vi "GVSView Pic Command Remove.vi"(10 "cCommand":T1) -> ()   [LabVIEW 2013]
uses:
  GVSView Global.vi
panel:
  out "Start_Positin 2":T2
  in  "ToolBar Click":bool
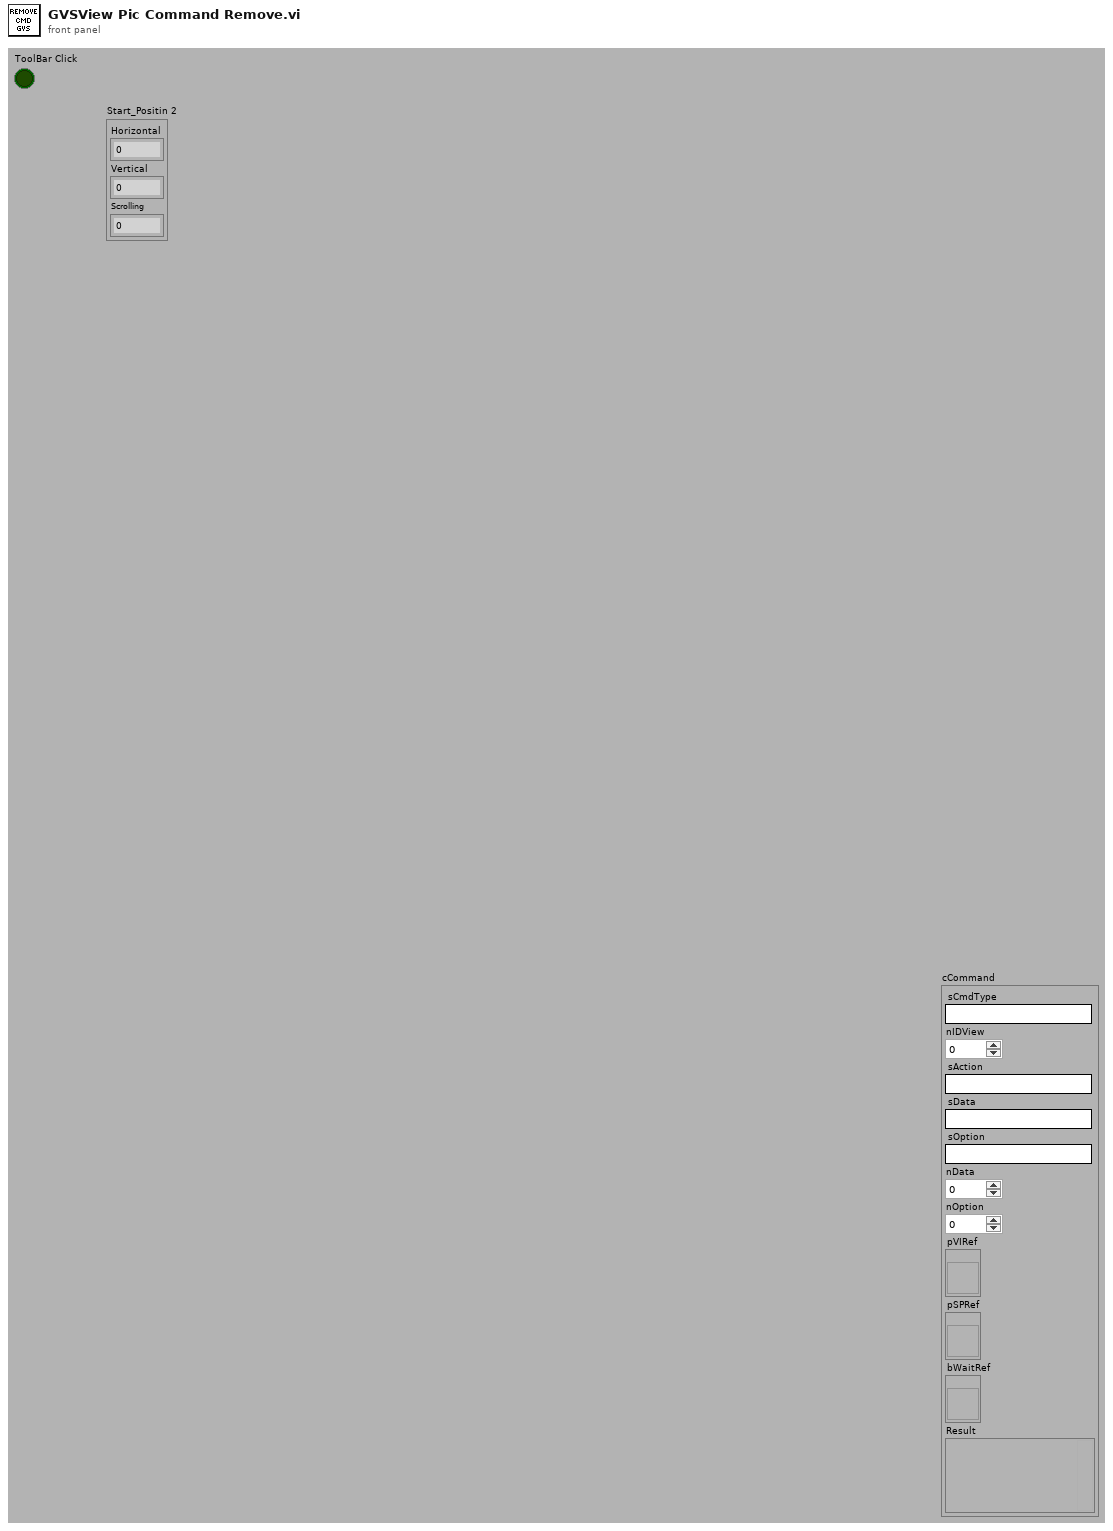
[diagram p1: front panel]
types:
  T1 = cluster{"sCmdType":string, "nIDView":i32, "sAction":string, "sData":string, "sOption":string, "nData":i32, "nOption":i32, "pVIRef":refnum<vi>, "pSPRef":refnum<vi>, "bWaitRef":refnum<vi>, "Result":variant}
  T2 = cluster{"Horizontal":i32, "Vertical":i32, "Scrolling":i32}
  T3 = cluster{"sCmdType":string, "nIDView":i32, "sAction":string, "sData":string, "sOption":string, "nData":i32, "nOption":i32, "pVIRef":refnum<vi>, "pSPRef":refnum<vi>, "bWaitRef":refnum<vi>, "Result":variant}[]
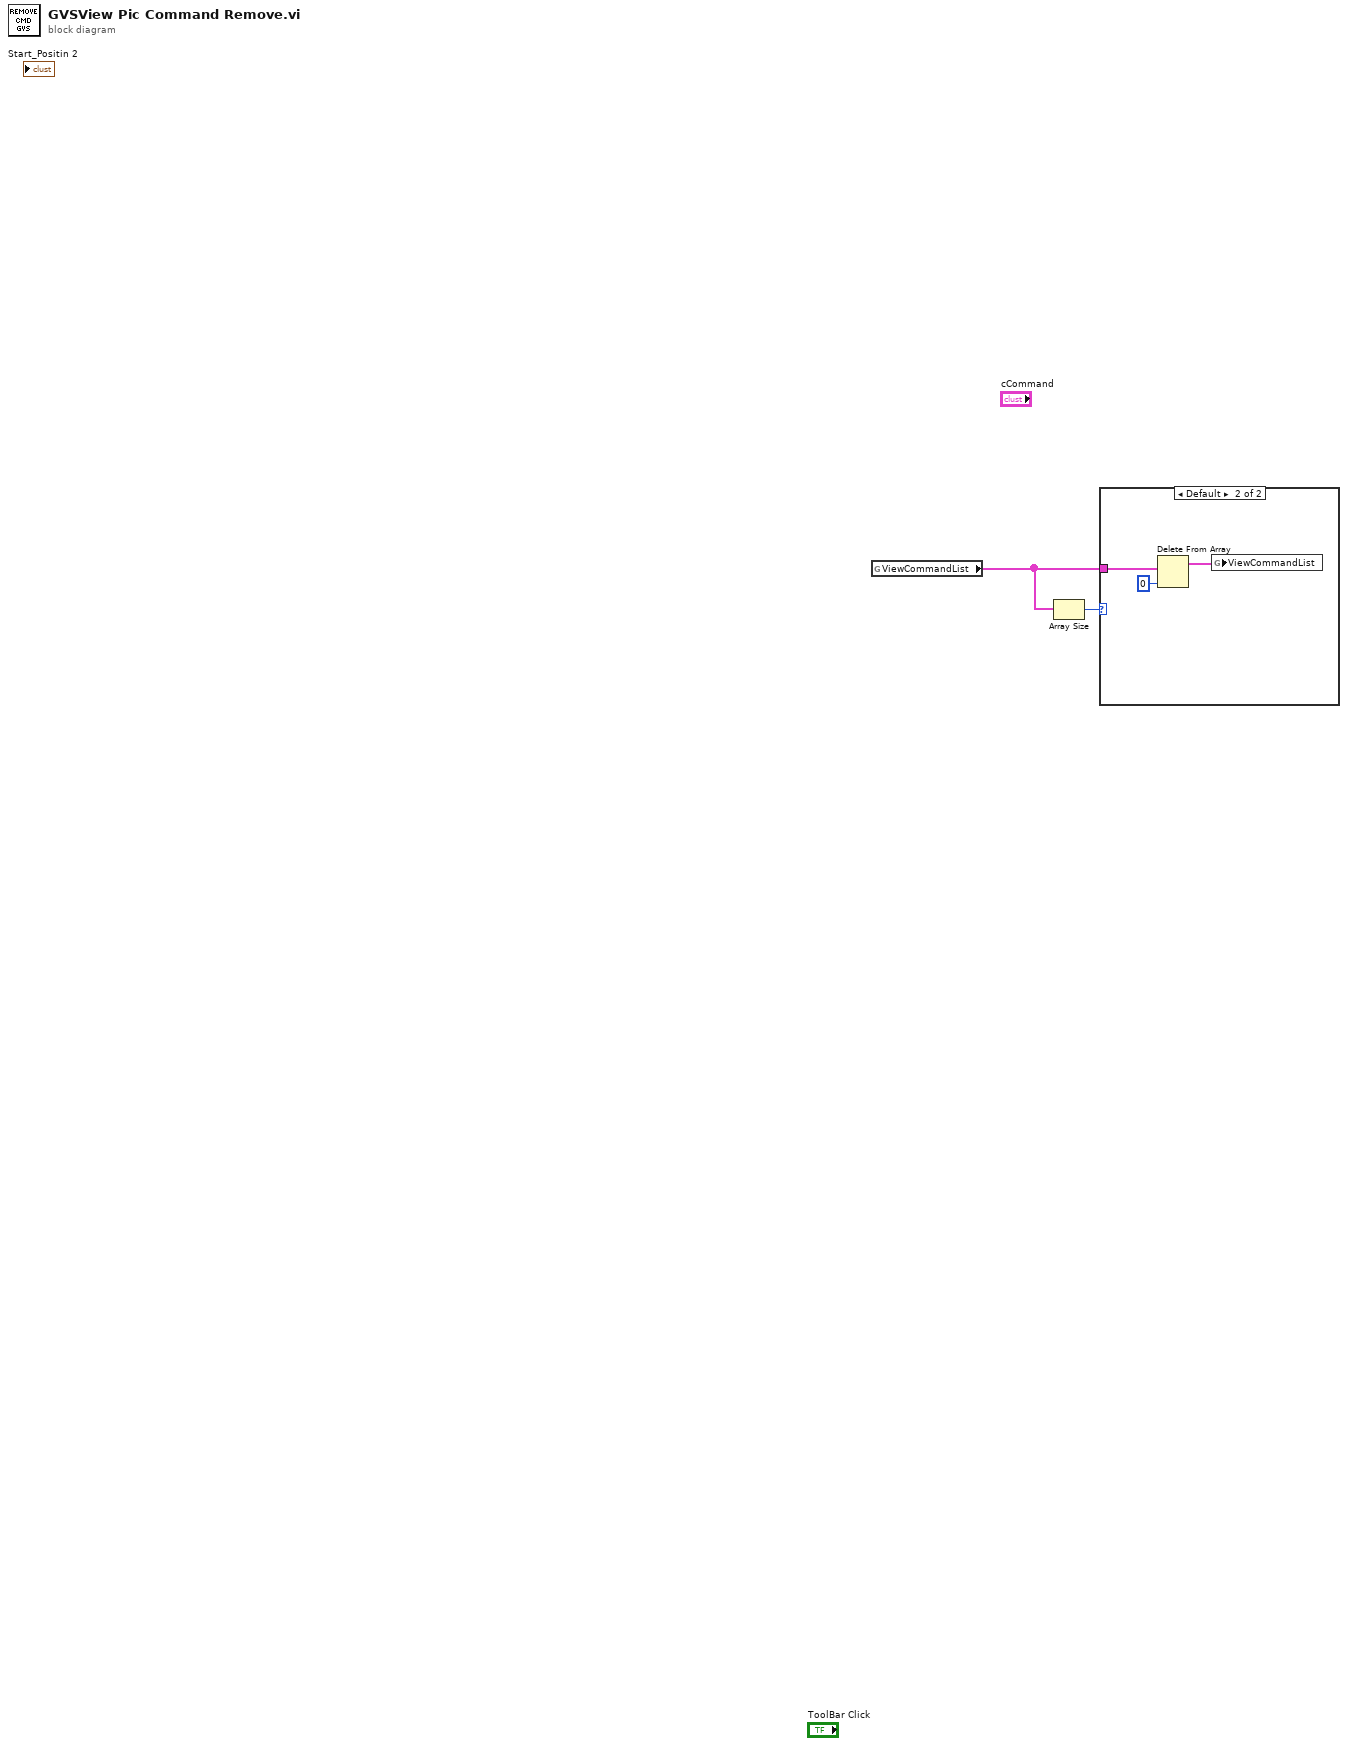
[diagram p0: block diagram]
diagram:
  n1 = global read "GVSView Global.vi" "ViewCommandList"() -> (w1:T3)
  n2 = Array Size(array=w1) -> (size(s)=w2:i32)
  n3 = case shown="Default" w2 {
    tunnel: w1 -> [_ w4]
    frame 0 {
    }
    frame Default {
      n4 = Delete From Array(array=w4, index=0) -> (array with subset deleted=w3:T3)  [unwired: 1 in, 1 out]
      n5 = global write "GVSView Global.vi" "ViewCommandList"(w3) -> ()
    }
  }
